vi "MessageCinematics.vi"(11 "Robot":T1={"id"=0, "function"=enum."Attacker", "x"=0.0, "y"=0.0, "orientation"=0.0, "v_tangent"=0.0, "v_normal"=0.0, "v_ang"=0.0, "kick_x"=0.0, "kick_z"=0.0, "dribble"=FALSE, "Timestamp"=timestamp(0 s since 1904-01-01), "estimatives"={"est_v_tangent"=0.0, "est_v_normal"=0.0, "est_vx"=0.0, "est_vy"=0.0, "Pos Robot Est"=[]}, "dest_x_kick"=0.0, "dest_y_kick"=0.0, "Gap Coord"=[], "States"=enum."GoToTangent", "Path "=[], "Path  Smooth"=[], "Dest"=[]}) -> (1 "Array":u8[](array[numeric]))   [LabVIEW 2017]
uses:
  Core/AI Robot.ctl
  Intel/Functions Enum.ctl
  Intel/AttackerStates.ctl
  Path Planning/RRT/PathDests.ctl
  Path Planning/RRT/PathDest.ctl
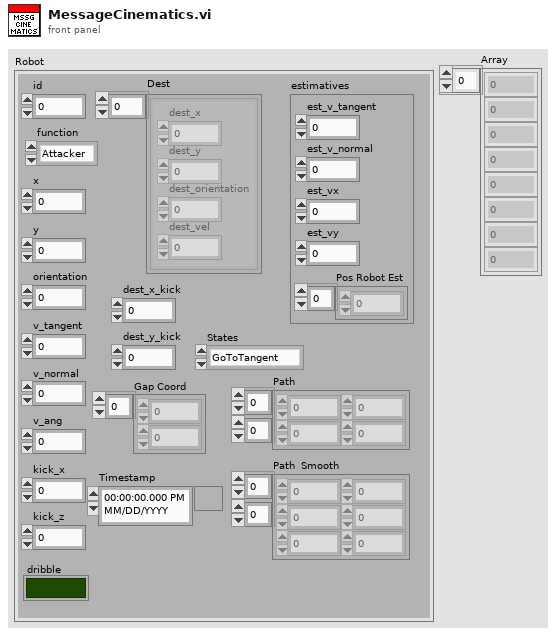
[diagram p1: front panel]
types:
  T1 = typedef "AI Robot.ctl" = cluster{"id":u32, "function":T2, "x":dbl, "y":dbl, "orientation":dbl, "v_tangent":dbl, "v_normal":dbl, "v_ang":dbl, "kick_x":dbl, "kick_z":dbl, "dribble":bool, "Timestamp":timestamp, "estimatives":cluster{"est_v_tangent":dbl, "est_v_normal":dbl, "est_vx":dbl, "est_vy":dbl, "Pos Robot Est":dbl[]}, "dest_x_kick":dbl, "dest_y_kick":dbl, "Gap Coord":dbl[], "States":T3, "Path ":dbl[][], "Path  Smooth":dbl[][], "Dest":T4}
  T2 = typedef "Functions Enum.ctl" = enum16{"Attacker", "Goalie", "Defender", "Striker", "Goto 0", "Dummy", "Kicker", "ZigZag"}
  T3 = typedef "AttackerStates.ctl" = enum16{"Pass", "GoToTangent", "BallGetting", "GoToKick", ""}
  T4 = typedef "PathDests.ctl" = T5[]
  T5 = typedef "PathDest.ctl" = cluster{"dest_x":dbl, "dest_y":dbl, "dest_orientation":dbl, "dest_vel":dbl}
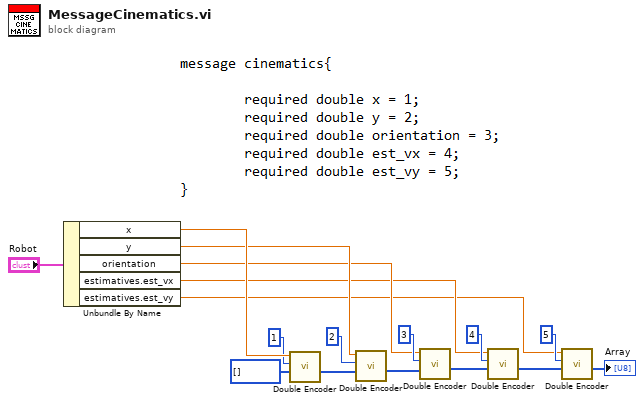
[diagram p0: block diagram]
diagram:
  n1 = Unbundle By Name("Robot") -> ("x"=w16:dbl, "y"=w6:dbl, "orientation"=w5:dbl, "estimatives.est_vx"=w4:dbl, "estimatives.est_vy"=w3:dbl)
  n2 = call "Double Encoder.vi"("Array In"=u8[] [], "Key"=u32 1, "Value"=w16) -> ("Array"=w13:u8[])  [unwired: 8 in]
  n3 = call "Double Encoder.vi"("Array In"=w13, "Key"=u32 2, "Value"=w6) -> ("Array"=w11:u8[])  [unwired: 8 in]
  n4 = call "Double Encoder.vi"("Array In"=w11, "Key"=u32 3, "Value"=w5) -> ("Array"=w9:u8[])  [unwired: 8 in]
  n5 = call "Double Encoder.vi"("Array In"=w9, "Key"=u32 4, "Value"=w4) -> ("Array"=w7:u8[])  [unwired: 8 in]
  n6 = call "Double Encoder.vi"("Array In"=w7, "Key"=u32 5, "Value"=w3) -> ("Array"=→"Array":u8[])  [unwired: 8 in]
